vi "Constructor.vi"(8 "error in":errorcluster, 11 "PID Detector in":refnum<class "INL PID.lvclass">) -> (0 "error out":errorcluster, 2 "init":bool, 3 "PID Detector out":refnum<class "INL PID.lvclass">)   [LabVIEW 2011, in "INL PID.lvclass"]
uses:
  INL PID.lvclass
  INL PID.lvclass/INL PID.ctl
  <vilib>/DAQmx/write.llb/DAQmx Write (Digital Bool 1Line 1Point).vi
  <vilib>/DAQmx/create/channels.llb/DAQmx Create Channel (CO-Pulse Generation-Time).vi
  <vilib>/DAQmx/create/channels.llb/DAQmx Create Channel (AI-Voltage-Basic).vi
  <vilib>/DAQmx/create/channels.llb/DAQmx Create Channel (DO-Digital Output).vi
  <vilib>/DAQmx/configure/timing.llb/DAQmx Timing (Sample Clock).vi
  <vilib>/DAQmx/configure/trigger.llb/DAQmx Start Trigger (Digital Edge).vi
  <vilib>/DAQmx/configure/timing.llb/DAQmx Timing (Implicit).vi
  <vilib>/DAQmx/miscellaneous.llb/DAQmx Fill In Error Info.vi
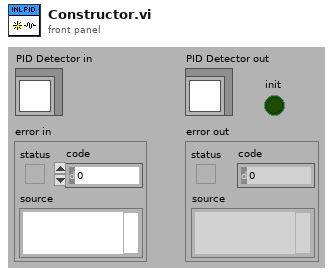
[diagram p1: front panel]
types:
  T1 = typedef "INL PID.lvclass/Integrator DAQmx Channels.ctl" = cluster{"V0":tag, "S1":tag, "S2":tag}
  T2 = typedef "INL PID.lvclass/Settings.ctl" = cluster{"Sampling Frequency":dbl, "Integration Time":dbl, "Integration Periods":u8, "Grid Voltage":dbl}
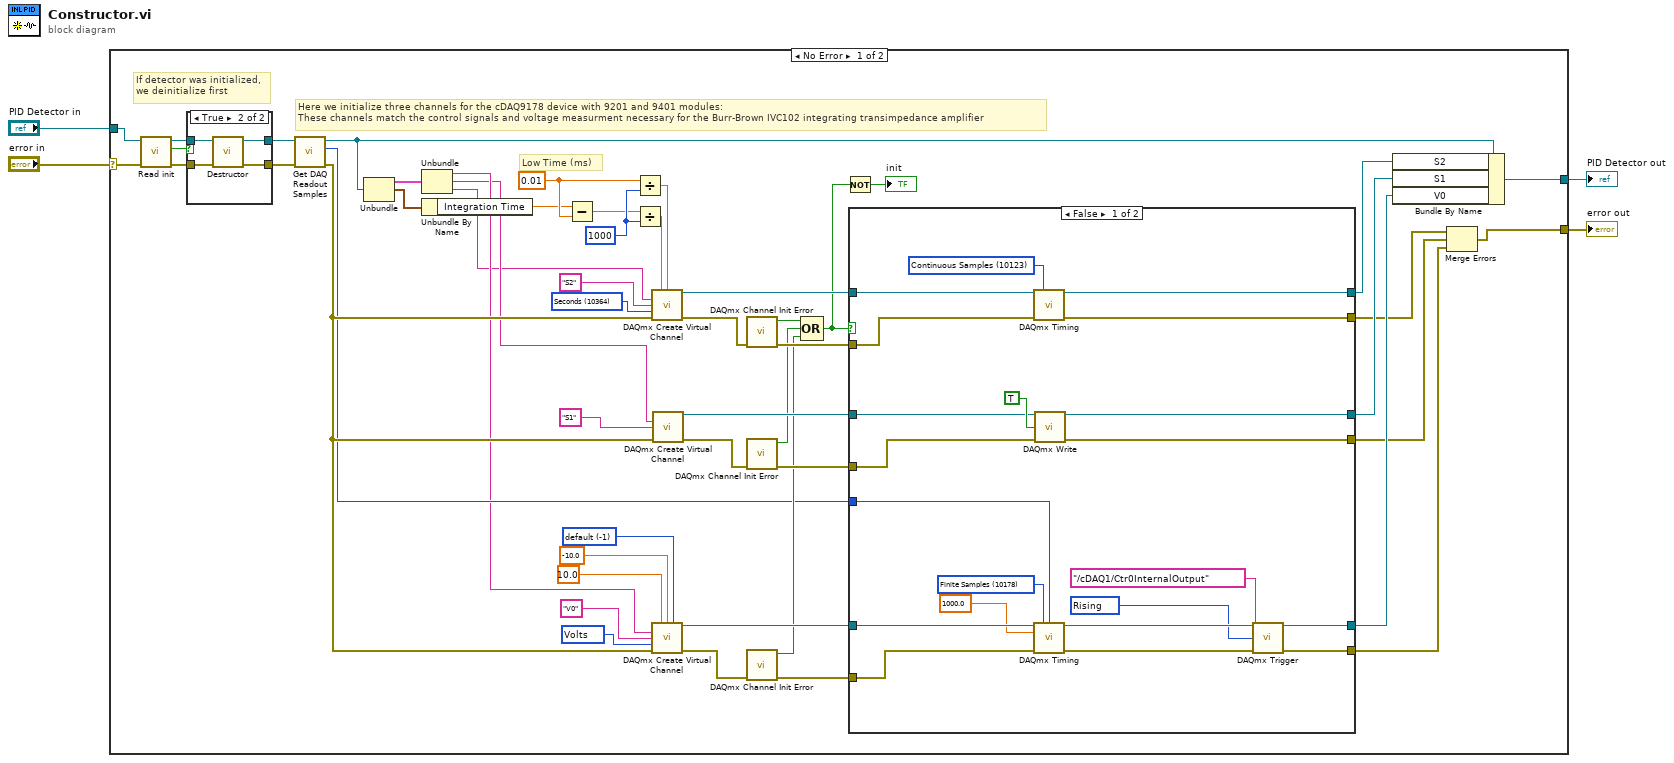
[diagram p0: block diagram]
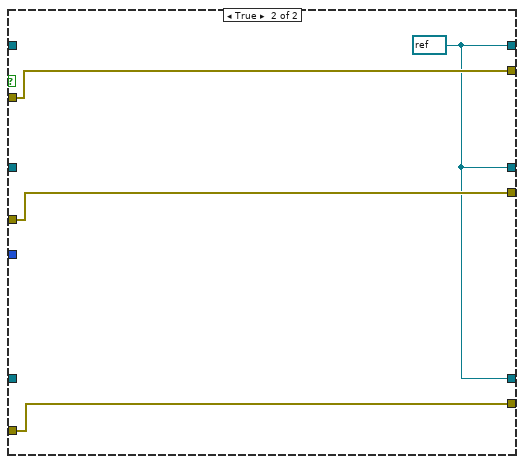
[diagram p2: hidden frame]
diagram:
  n1 = case shown="No Error" "error in" {
    selector: "error in" -> [w12 w88]
    tunnel: [w54 w88] -> w3
    tunnel: [w55 w87] -> w1
    tunnel: "PID Detector in" -> [w11 w87]
    frame No Error {
      w48 = -1 items=["default"=-1, "RSE"=10083, "NRSE"=10078, "Differential"=10106, "Pseudodifferential"=12529] ("input terminal configuration")
      w45 = 10348 items=["Volts"=10348, "From Custom Scale"=10065] ("V0 units")
      w49 = 10364 items=["Seconds"=10364] ("S2 units")
      w33 = 0.01 ("low time (ms)")
      w37 = 1000
      # "If detector was initialized,\nwe deinitialize first"
      # "Here we initialize three channels for the cDAQ9178 device with 9201 and 9401 modules:\nThese channels match the control signals and voltage measurment necessary for the Burr-Brown IVC102 integrating transimpedance amplifier"
      # "Low Time (ms)"
      n2 = call-dynamic "Read init.vi"("error in (no error)"=w12, "Detector in"=w11) -> ("error out"=w52:errorcluster, "init"=w51:bool, "Detector out"=w53:refnum<class "INL PID.lvclass">)  [unwired: 7 in]
      n3 = case shown="True" w51 {
        tunnel: w52 -> [w81 w85]
        tunnel: w53 -> [w82 w86]
        tunnel: [w82 w84] -> w10
        tunnel: [w81 w83] -> w9
        frame False {
        }
        frame True {
          n4 = call-dynamic "Destructor.vi"("error in"=w85, "PID in"=w86) -> ("error out"=w83:errorcluster, "PID out"=w84:refnum<class "INL PID.lvclass">)  [unwired: 8 in]
        }
      }
      n5 = call-dynamic "Get DAQ Readout Samples.vi"("error in"=w9, "INL PID in"=w10) -> ("error out"=w30:errorcluster, "ReadOut Samples"=w8:i32, "INL PID out"=w29:refnum<class "INL PID.lvclass">)  [unwired: 7 in]
      n6 = Unbundle(w29) -> (w31:T1, w14:T2)  [unwired: 1 out]
      n7 = Unbundle(w31) -> ("V0"=w7:tag, "S1"=w6:tag, "S2"=w5:tag)
      n8 = Unbundle By Name(w14) -> ("Integration Time"=w13:dbl)
      n9 = Subtract(x=w13, y=w33) -> (x-y=w32:dbl)
      n10 = Divide(x=w33, y=w37) -> (x/y=w39:dbl)
      n11 = Divide(x=w32, y=w37) -> (x/y=w38:dbl)
      n12 = call-poly <vilib>:"DAQmx Create Virtual Channel.vi"("high time"=w38, "low time"=w39, "counter"=w5, "name to assign"="S2", "units"=w49, "error in"=w30) -> ("task out"=w50:refnum<k21>, "error out"=w28:errorcluster)  [unwired: 8 in]
      n13 = call-poly <vilib>:"DAQmx Create Virtual Channel.vi"("maximum value"=10.0, "minimum value"=-10.0, "input terminal configuration"=w48, "physical channels"=w7, "name to assign"="V0", "units"=w45, "error in"=w30) -> ("task out"=w44:refnum<k21>, "error out"=w25:errorcluster)  [unwired: 7 in]
      n14 = call-poly <vilib>:"DAQmx Create Virtual Channel.vi"("lines"=w6, "name to assign"="S1", "error in"=w30) -> ("task out"=w43:refnum<k21>, "error out"=w26:errorcluster)  [unwired: 11 in]
      n15 = call "DAQmx Channel Init Error.vi"("error in"=w28) -> ("error out"=w27:errorcluster, "channel init error?"=w22:bool)  [unwired: 9 in]
      n16 = call "DAQmx Channel Init Error.vi"("error in"=w26) -> ("error out"=w24:errorcluster, "channel init error?"=w21:bool)  [unwired: 9 in]
      n17 = call "DAQmx Channel Init Error.vi"("error in"=w25) -> ("error out"=w23:errorcluster, "channel init error?"=w20:bool)  [unwired: 9 in]
      n18 = Compound Arithmetic op=OR(w22, w21, w20) -> (w15:bool)
      n19 = Not(x=w15) -> (.not. x?=→"init":bool)
      n20 = case shown="False" w15 {
        tunnel: w50 -> [w76 _]
        tunnel: w44 -> [w74 _]
        tunnel: w43 -> [w70 _]
        tunnel: [w65 w77] -> w36
        tunnel: [w64 w77] -> w35
        tunnel: [w63 w77] -> w34
        tunnel: w27 -> [w62 w80]
        tunnel: w24 -> [w61 w79]
        tunnel: w23 -> [w60 w78]
        tunnel: [w59 w80] -> w19
        tunnel: [w58 w79] -> w18
        tunnel: [w57 w78] -> w17
        tunnel: w8 -> [w56 _]
        frame False {
          w75 = 10123 items=["Finite Samples"=10178, "Continuous Samples"=10123, "Hardware Timed Single Point"=12522] ("sample mode")
          w67 = 10280 items=["Rising"=10280, "Falling"=10171] ("edge")
          w73 = 10178 items=["Finite Samples"=10178, "Continuous Samples"=10123, "Hardware Timed Single Point"=12522] ("sample mode")
          n21 = call-poly <vilib>:"DAQmx Timing.vi"("task/channels in"=w76, "sample mode"=w75, "error in"=w62) -> ("task out"=w65:refnum<k21>, "error out"=w59:errorcluster)  [unwired: 11 in]
          n22 = call-poly <vilib>:"DAQmx Timing.vi"("task/channels in"=w74, "sample mode"=w73, "samples per channel"=w56, "rate"=1000.0, "error in"=w60) -> ("task out"=w69:refnum<k21>, "error out"=w68:errorcluster)  [unwired: 9 in]
          n23 = call-poly <vilib>:"DAQmx Write.vi"("task/channels in"=w70, "data"=TRUE, "error in"=w61) -> ("task out"=w64:refnum<k21>, "error out"=w58:errorcluster)  [unwired: 10 in, 1 out]
          n24 = call-poly <vilib>:"DAQmx Trigger.vi"("task/channels in"=w69, "source"=tag "/cDAQ1/Ctr0InternalOutput", "edge"=w67, "error in"=w68) -> ("task out"=w63:refnum<k21>, "error out"=w57:errorcluster)  [unwired: 10 in]
        }
        frame True {
          w77 = refnum<k21> refnum ("task out")
        }
      }
      n25 = Bundle By Name(cluster=w29, "S2"=w36, "S1"=w35, "V0"=w34) -> (w55:refnum<class "INL PID.lvclass">)
      n26 = Merge Errors(w19, w18, w17) -> (w54:errorcluster)
    }
    frame Error {
    }
  }
  "error out" <- w3
  "PID Detector out" <- w1
